vi "plugins_unload.vi"(4 "error in (no error)":errorcluster, 5 "Plugins":T1(array[cluster]), 6 "Sub Panel":refnum<vi>, 7 "Plugin Chooser":refnum<vi>) -> (2 "Sub Panel Out":refnum<vi>, 3 "Plugin Chooser Out":refnum<vi>)   [LabVIEW 2015]
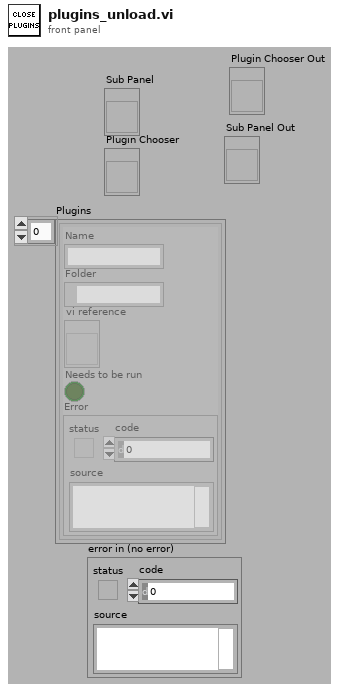
[diagram p1: front panel]
types:
  T1 = cluster{"Name":string, "Folder":path, "vi reference":refnum<vi>, "Needs to be run":bool, "Error":errorcluster}[]
  T2 = enum32{"Bad", "Idle", "Run top level", "Running"}
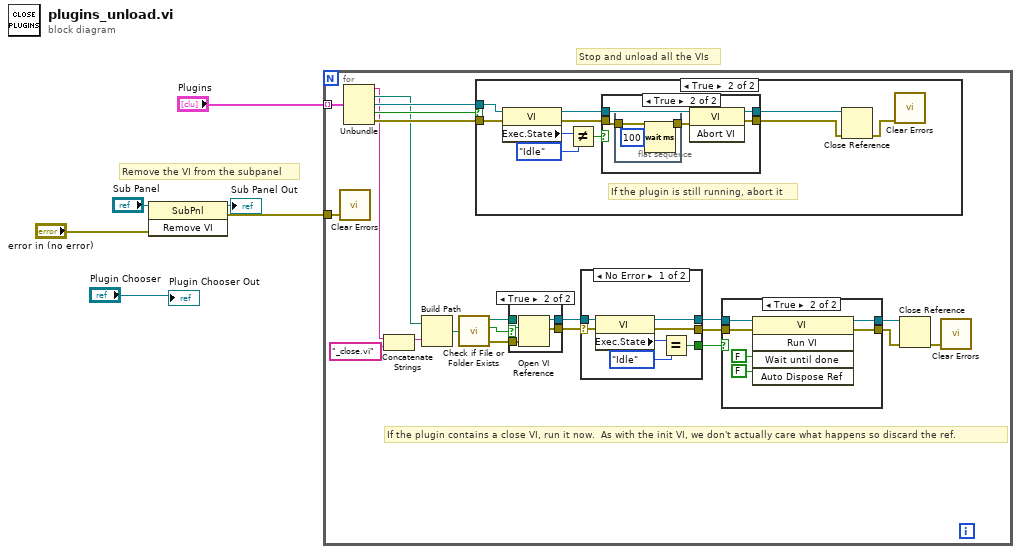
[diagram p0: block diagram]
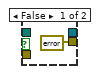
[diagram p3: hidden frame]
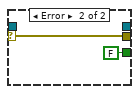
[diagram p4: hidden frame]
diagram:
  # "Stop and unload all the VIs"
  # "Remove the VI from the subpanel"
  n1 = invoke class="SubPnl" method="Remove VI"(reference="Sub Panel", error in="error in (no error)") -> (reference out=→"Sub Panel Out":refnum<vi>, error out=w1:errorcluster)  [unwired: 1 in, 1 out]
  n2 = for {
    tunnel: "Plugins" -> [w27] mode=indexing
    tunnel: w1 -> [w7]
    # "If the plugin contains a close VI, run it now.  As with the init VI, we don't actually care what happens so discard the ref."
    n3 = call <vilib>:"Clear Errors.vi"("error in (no error)"=w7) -> ()  [unwired: 5 in, 2 out]
    n4 = Unbundle(w27) -> ("Name"=w8:string, "Folder"=w10:path, "vi reference"=w11:refnum<vi>, "Needs to be run"=w25:bool, "Error"=w26:errorcluster)
    n5 = Concatenate Strings(w8, "_close.vi" ("string")) -> (w20:string)
    n6 = Build Path(base path=w10, name or relative path=w20) -> (appended path=w12:path)
    n7 = call <vilib>:"Check if File or Folder Exists.vi"("path"=w12) -> ("error out"=w18:errorcluster, "file or folder exists?"=w24:bool, "dup path"=w21:path)  [unwired: 8 in]
    n8 = case shown="True" w25 {
      tunnel: w11 -> [_ w54]
      tunnel: w26 -> [_ w53]
      frame False {
      }
      frame True {
        # "If the plugin is still running, abort it"
        n9 = property class="VI"(reference=w54, error in=w53) -> (reference out=w56:refnum<vi>, error out=w55:errorcluster, "Exec.State"=w59:T2)
        n10 = Not Equal?(x=w59, y=T2."Idle") -> (x != y?=w57:bool)
        n11 = case shown="True" w57 {
          tunnel: w56 -> [w61 w66]
          tunnel: w55 -> [w60 w63]
          tunnel: [w60 w65] -> w51
          tunnel: [w61 w64] -> w52
          frame False {
          }
          frame True {
            n12 = flat-sequence {
              tunnel: w63 -> [w67]
              tunnel: [w67] -> w62
              frame #0 {
                n13 = Wait (ms)(milliseconds to wait=u32 100) -> ()  [unwired: 1 out]
              }
            }
            n14 = invoke class="VI" method="Abort VI"(reference=w66, error in=w62) -> (reference out=w64:refnum<vi>, error out=w65:errorcluster)  [unwired: 1 in, 1 out]
          }
        }
        n15 = Close Reference(reference=w52, error in (no error)=w51) -> (error out=w50:errorcluster)
        n16 = call <vilib>:"Clear Errors.vi"("error in (no error)"=w50) -> ()  [unwired: 5 in, 2 out]
      }
    }
    n17 = case shown="True" w24 {
      tunnel: w21 -> [_ w40]
      tunnel: [_ w39] -> w22
      tunnel: [errorcluster {"status"=TRUE, "code"=0, "source"=""} ("error out") w38] -> w23
      tunnel: w18 -> [_ w37]
      frame False {
      }
      frame True {
        n18 = Open VI Reference(vi path=w40, error in (no error)=w37) -> (vi reference=w39:refnum<vi>, error out=w38:errorcluster)  [unwired: 4 in]
      }
    }
    n19 = case shown="No Error" w23 {
      selector: w23 -> [w42 w48]
      tunnel: w22 -> [w41 _]
      tunnel: [w47 _] -> w15
      tunnel: [w46 FALSE] -> w17
      tunnel: [w43 w48] -> w16
      frame No Error {
        n20 = property class="VI"(reference=w41, error in=w42) -> (reference out=w47:refnum<vi>, error out=w43:errorcluster, "Exec.State"=w45:T2)
        n21 = Equal?(x=w45, y=T2."Idle" ("Execution:State")) -> (x = y?=w46:bool)
      }
      frame Error {
      }
    }
    n22 = case shown="True" w17 {
      tunnel: w15 -> [w29 w35]
      tunnel: w16 -> [w28 w34]
      tunnel: [w29 w31] -> w14
      tunnel: [w28 w30] -> w13
      frame False {
      }
      frame True {
        n23 = invoke class="VI" method="Run VI"(reference=w35, error in=w34, "Wait until done"=FALSE ("Wait Until Done"), "Auto Dispose Ref"=FALSE ("Auto Dispose Reference")) -> (reference out=w31:refnum<vi>, error out=w30:errorcluster)  [unwired: 1 in, 3 out]
      }
    }
    n24 = Close Reference(reference=w14, error in (no error)=w13) -> (error out=w9:errorcluster)
    n25 = call <vilib>:"Clear Errors.vi"("error in (no error)"=w9) -> ()  [unwired: 5 in, 2 out]
  }
  "Plugin Chooser Out" <- "Plugin Chooser"
